vi "Find and assign COM Ports_1.vi"(8 "error in (no error)":errorcluster) -> (0 "error out":errorcluster, 2 "Available COM Ports":refnum<visa-resource-name>[](array[refnum]), 3 "Assigned VISA Ports":T1(array[cluster]))   [LabVIEW 2018]
uses:
  <vilib>/Instr/_visa.llb/VISA Find Search Mode.ctl
  <vilib>/Instr/_visa.llb/VISA Configure Serial Port (Instr).vi
panel:
  out "Available USB Ports":refnum<visa-resource-name>[](array[refnum])
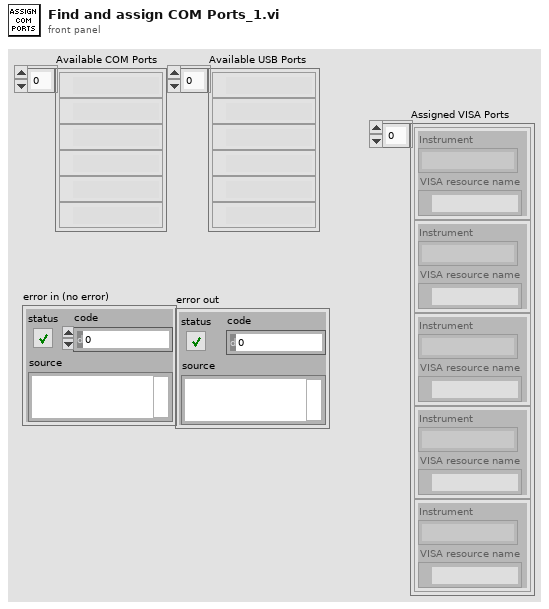
[diagram p1: front panel]
types:
  T1 = cluster{"Instrument":string, "VISA resource name":refnum<visa-resource-name>}[]
  T2 = enum16{"Switch", "SMU", "Vitrek", "Valhalla", "Stop"}
  T3 = typedef "VISA Find Search Mode.ctl" = u32
  T4 = cluster{"Instrument":string, "VISA resource name":refnum<visa-resource-name>}
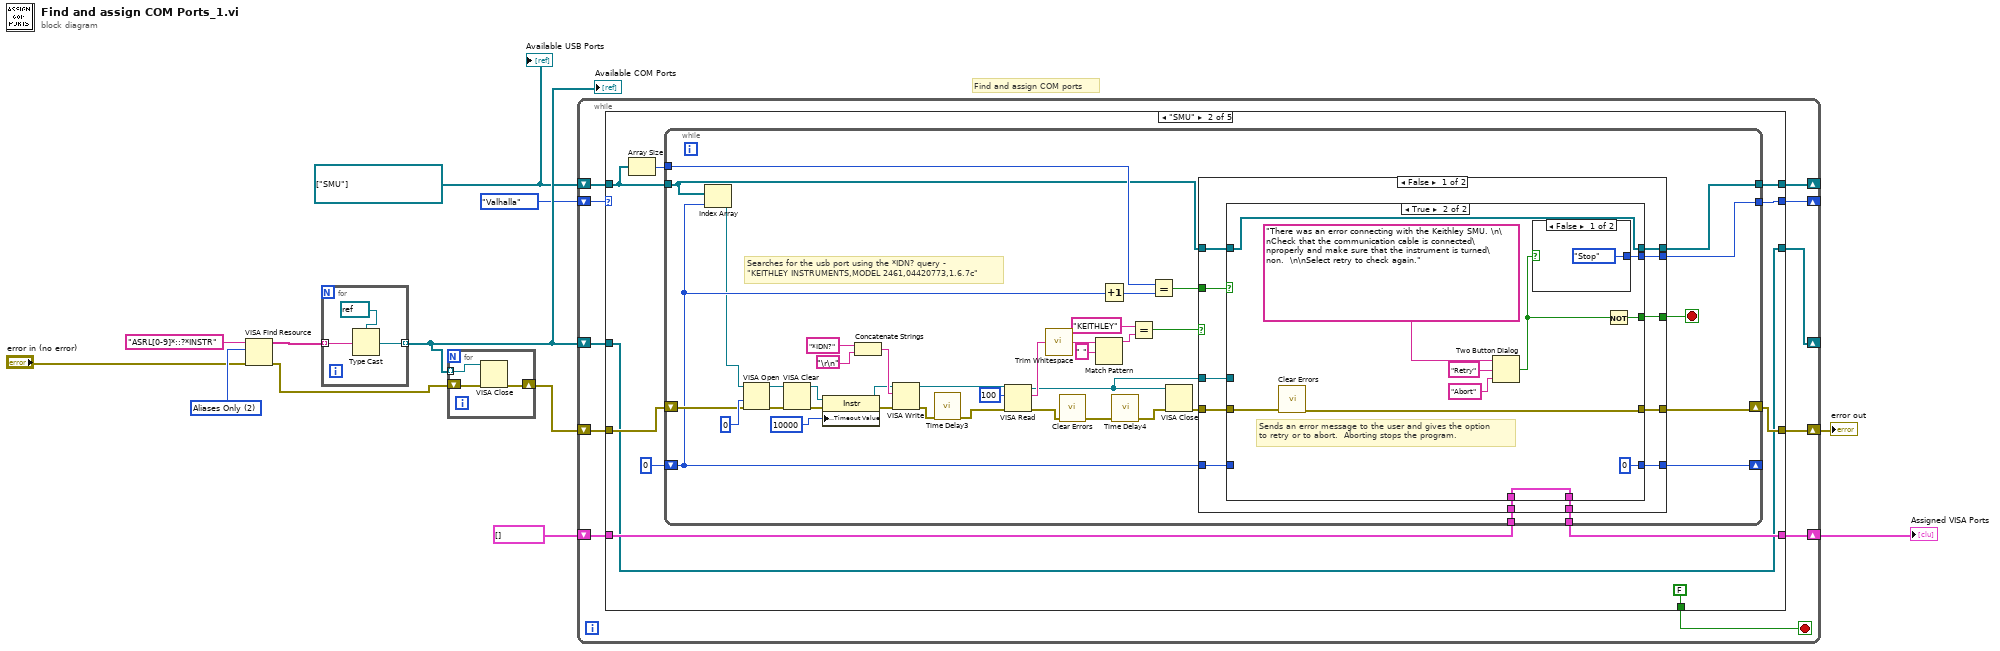
[diagram p0: block diagram]
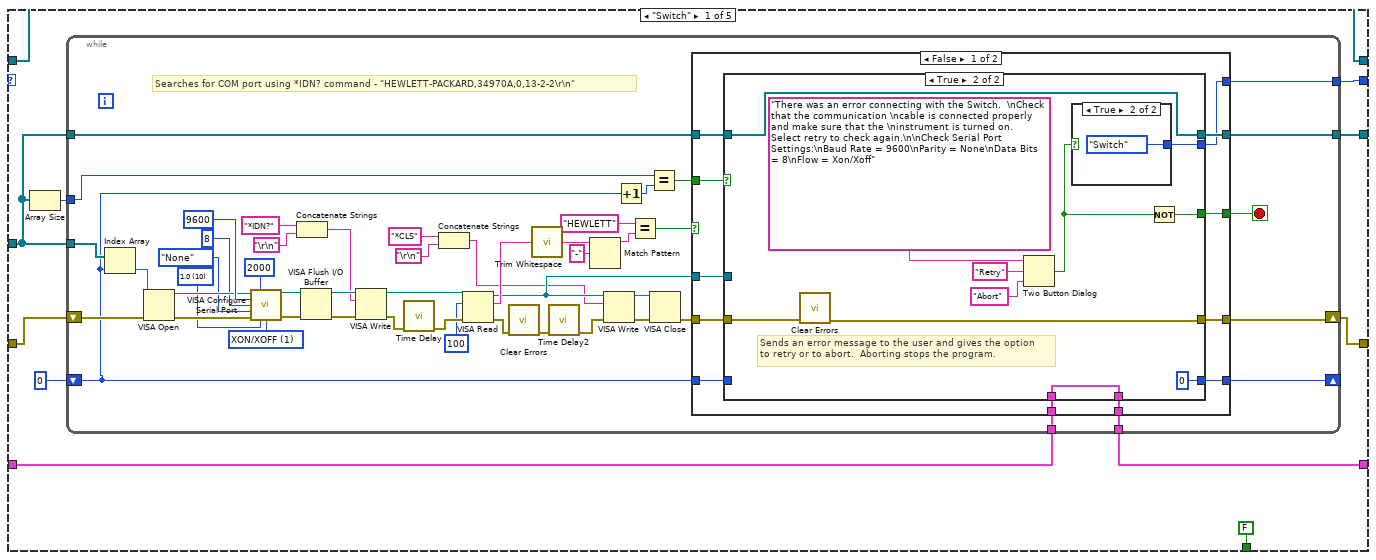
[diagram p2: hidden frame]
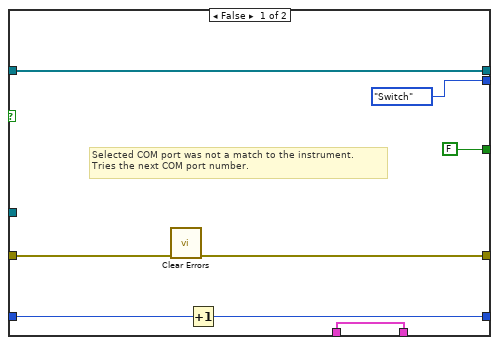
[diagram p3: hidden frame]
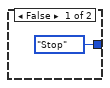
[diagram p4: hidden frame]
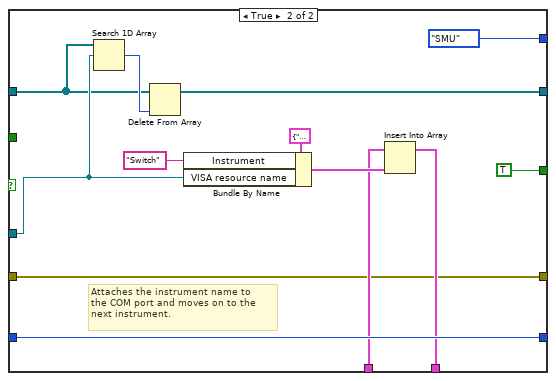
[diagram p5: hidden frame]
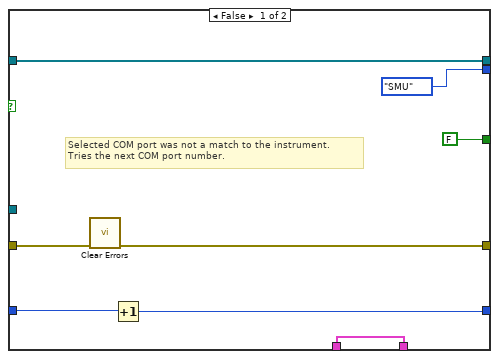
[diagram p6: hidden frame]
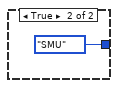
[diagram p7: hidden frame]
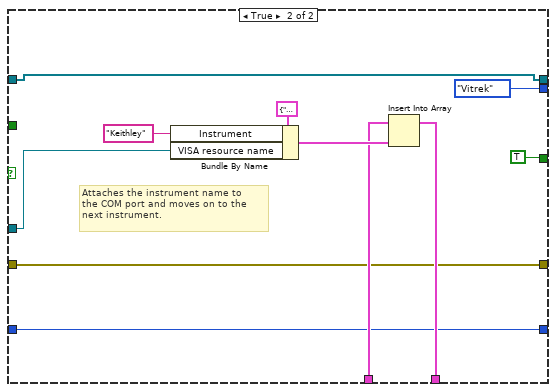
[diagram p8: hidden frame]
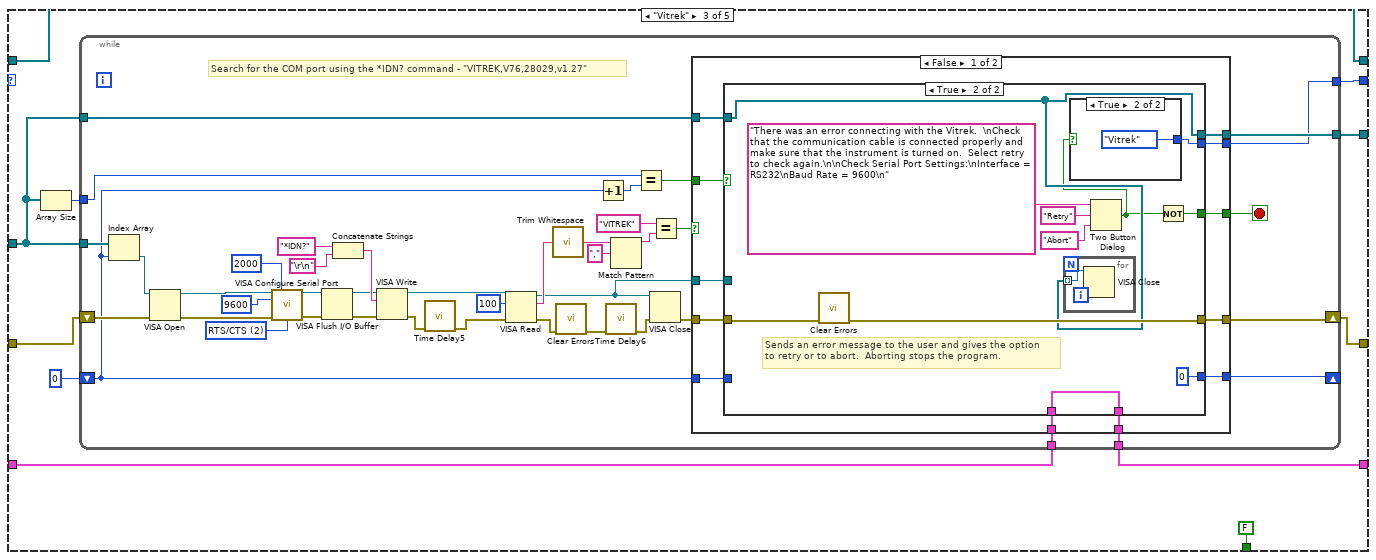
[diagram p9: hidden frame]
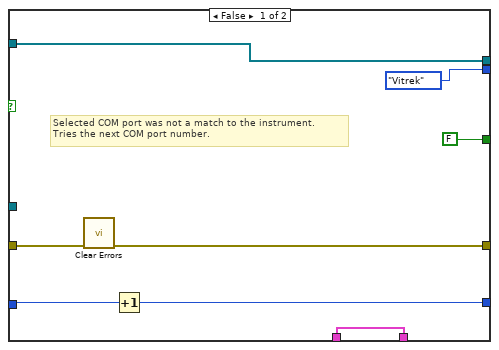
[diagram p10: hidden frame]
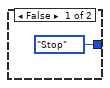
[diagram p11: hidden frame]
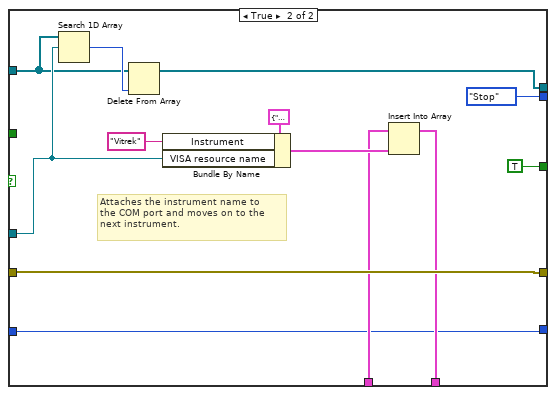
[diagram p12: hidden frame]
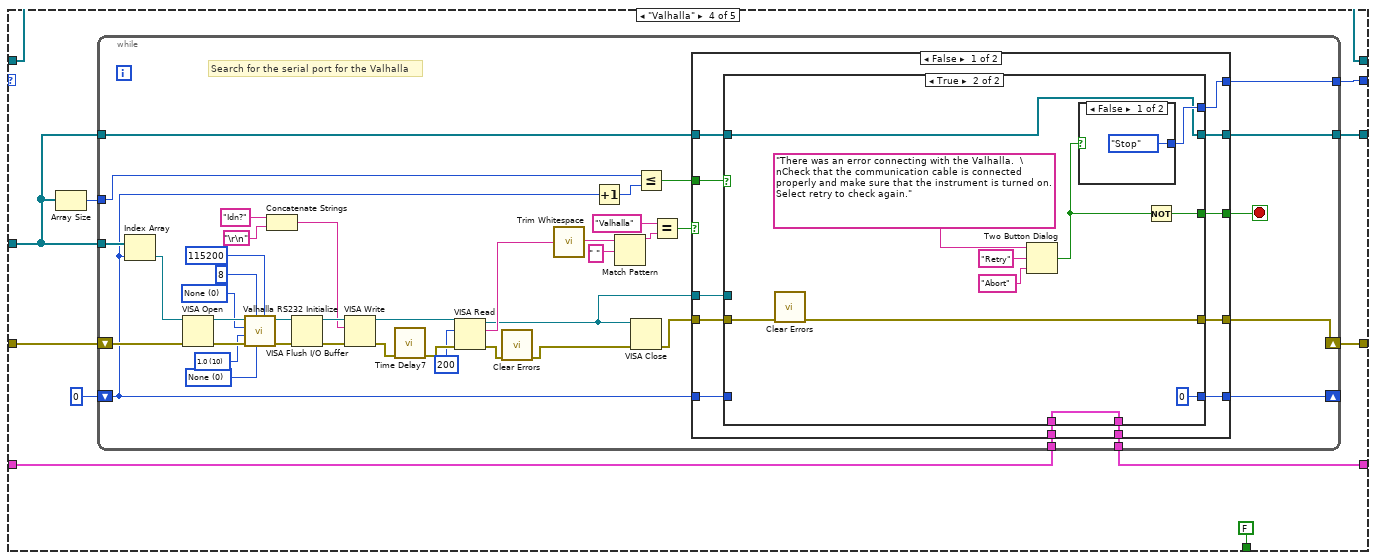
[diagram p13: hidden frame]
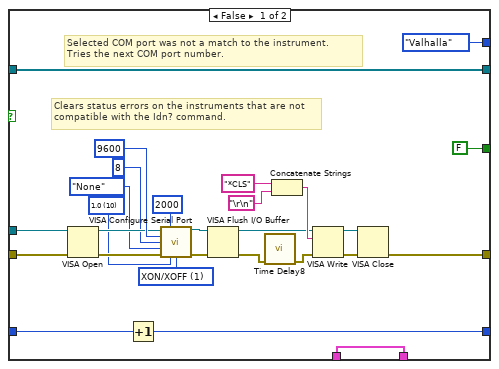
[diagram p14: hidden frame]
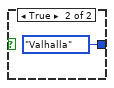
[diagram p15: hidden frame]
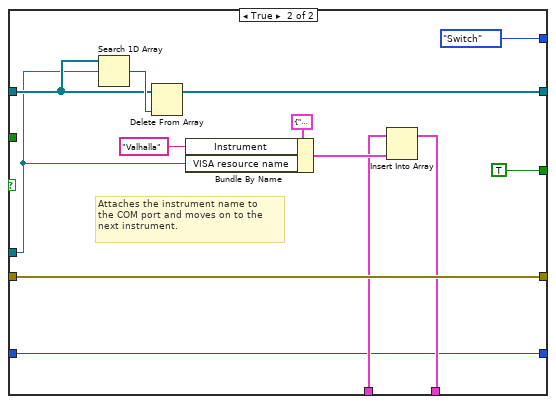
[diagram p16: hidden frame]
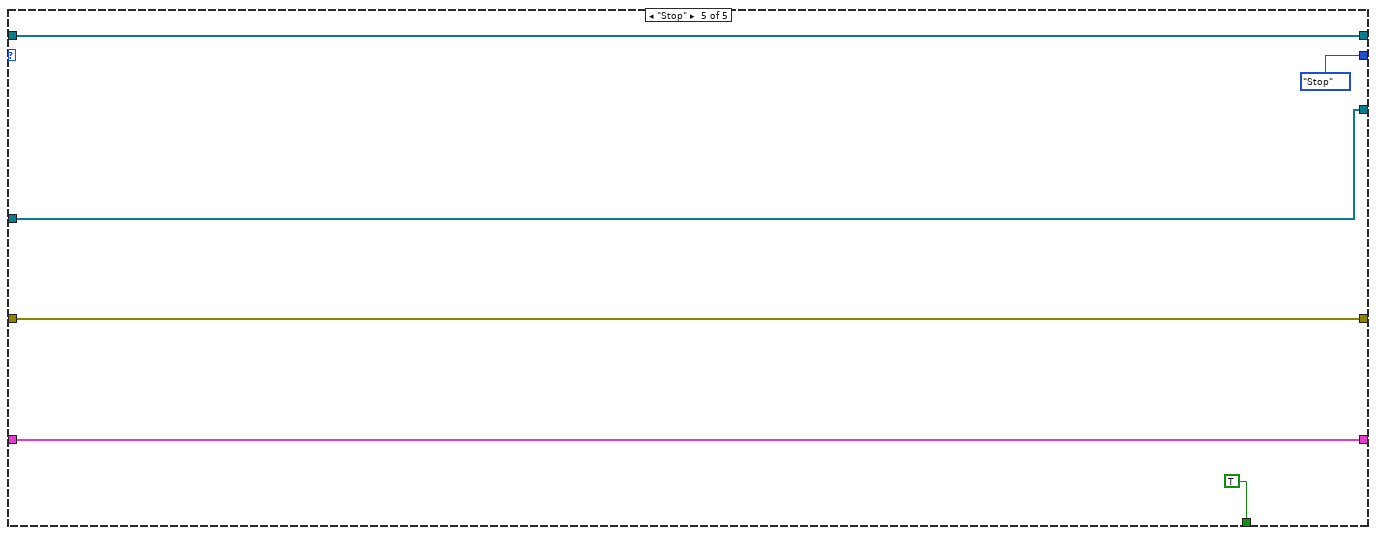
[diagram p17: hidden frame]
diagram:
  w1 = refnum<visa-resource-name>[] ["SMU"] ("Array")
  w7 = T3 2 items=["Canonical Names Only"=0, "Aliases Only"=2, "Include Matching Aliases"=3, "Include All Aliases"=4] ("Search Mode")
  # "Find and assign COM ports"
  n1 = VISA Find Resource(8:"error in (no error)", 10:w7, 11:"ASRL[0-9]*::?*INSTR" ("expression (\"?*\")")) -> (0:w3:errorcluster, 3:w8:string[])  [unwired: 1 out]
  n2 = for {
    tunnel: w8 -> [w14] mode=indexing
    tunnel: [w13] -> w12 mode=indexing
    n3 = Type Cast(type=refnum<visa-resource-name> refnum ("VISA resource name"), x=w14) -> (*(type *) &x=w13:refnum<visa-resource-name>)
  }
  "Available COM Ports" <- w12
  n4 = for {
    tunnel: w12 -> [w18] mode=indexing
    shift-right: [w16] -> w2
    shift-left: w3 -> [w17]
    n5 = VISA Close(VISA resource name=w18, error in (no error)=w17) -> (error out=w16:errorcluster)
  }
  n6 = while {
    shift-right: [w26] -> _
    shift-left: T2."Valhalla" ("Enum") -> [w28]
    shift-right: [w27] -> w11
    shift-left: T1 [] -> [w25]
    shift-right: [w24] -> _
    shift-left: w12 -> [w29]
    shift-right: [w22] -> w4
    shift-left: w2 -> [w23]
    shift-right: [w19] -> _
    shift-left: w1 -> [w20]
    stop <- w21 stop-if-true
    n7 = case shown="\"SMU\"" w28 {
      tunnel: [w33 w143 w235 w335 w456] -> w22
      tunnel: w29 -> [w37 w137 w239 w339 w454]
      tunnel: [w38 w146 w240 w340 w455] -> w27
      tunnel: [w35 w145 w237 w337 T2."Stop" ("Enum")] -> w26
      tunnel: w25 -> [w39 w147 w241 w341 w455]
      tunnel: [w36 w137 w238 w338 w454] -> w24
      tunnel: w23 -> [w34 w144 w236 w336 w456]
      tunnel: [FALSE FALSE FALSE FALSE TRUE] -> w21
      tunnel: w20 -> [w30 w140 w232 w332 w451]
      tunnel: [w30 w138 w232 w332 w451] -> w19
      frame "Switch" {
        n8 = Array Size(array=w37) -> (size(s)=w40:i32)
        n9 = while {
          tunnel: w37 -> [w46]
          tunnel: w40 -> [w81]
          tunnel: w39 -> [w72]
          tunnel: [w71] -> w38
          tunnel: w37 -> [w70]
          tunnel: [w69] -> w36
          tunnel: [w67] -> w35
          shift-right: [w66] -> w33
          shift-left: w34 -> [w65]
          shift-right: [w44] -> _
          shift-left: 0 -> [w41]
          stop <- w73 stop-if-true
          w60 = u16 10 items=["1.0"=10, "1.5"=15, "2.0"=20] ("stop bits (10: 1 bit)")
          w90 = u16 1 items=["None", "XON/XOFF", "RTS/CTS", "XON/XOFF & RTS/CTS", "DTR/DSR", "XON/XOFF & DTR/DSR"] ("flow control (0:none)")
          # "Searches for COM port using *IDN? command - \"HEWLETT-PACKARD,34970A,0,13-2-2\\r\\n\""
          n10 = Index Array(array=w46, index=w41) -> (element=w45:refnum<visa-resource-name>)
          n11 = VISA Open(error in (no error)=w65, VISA resource name=w45) -> (VISA resource name=w63:refnum<visa-resource-name>, error out=w64:errorcluster)  [unwired: 3 in]
          n12 = call-poly "VISA Configure Serial Port"("VISA resource name"=w63, "timeout (10sec)"=u32 2000, "baud rate (9600)"=u32 9600, "data bits (8)"=u16 8, "parity (0:none)"=enum16{"None", "Odd", "Even", "Mark", "Space"}."None", "error in (no error)"=w64, "stop bits (10: 1 bit)"=w60, "flow control (0:none)"=w90) -> ("VISA resource name out"=w77:refnum<visa-resource-name>, "error out"=w75:errorcluster)  [unwired: 6 in]
          n13 = Concatenate Strings("*IDN?" ("write buffer"), "\r\n") -> (w56:string)
          n14 = VISA Flush I/O Buffer(VISA resource name=w77, error in (no error)=w75) -> (VISA resource name out=w76:refnum<visa-resource-name>, error out=w74:errorcluster)  [unwired: 1 in]
          n15 = VISA Write(VISA resource name=w76, write buffer=w56, error in (no error)=w74) -> (VISA resource name out=w87:refnum<visa-resource-name>, error out=w88:errorcluster)  [unwired: 1 out]
          n16 = call "Time Delay"("error in (no error)"=w88) -> ("error out"=w86:errorcluster)  [unwired: 10 in]
          n17 = Concatenate Strings("*CLS" ("write buffer"), "\r\n") -> (w48:string)
          n18 = VISA Read(VISA resource name=w87, byte count=u32 100, error in (no error)=w86) -> (VISA resource name out=w50:refnum<visa-resource-name>, read buffer=w78:string, error out=w59:errorcluster)  [unwired: 1 out]
          n19 = call <vilib>:"Clear Errors.vi"("error in (no error)"=w59) -> ("error out"=w58:errorcluster)  [unwired: 5 in, 1 out]
          n20 = call <vilib>:"Trim Whitespace.vi"("string"=w78) -> ("trimmed string"=w80:string)  [unwired: 1 in]
          n21 = call "Time Delay2"("error in (no error)"=w58) -> ("error out"=w52:errorcluster)  [unwired: 10 in]
          n22 = Match Pattern(string=w80, regular expression="-") -> (before substring=w79:string)  [unwired: 1 in, 3 out]
          n23 = VISA Write(VISA resource name=w50, write buffer=w48, error in (no error)=w52) -> (VISA resource name out=w49:refnum<visa-resource-name>, error out=w51:errorcluster)  [unwired: 1 out]
          n24 = Increment(x=w41) -> (x+1=w47:i32)
          n25 = Equal?(x="HEWLETT", y=w79) -> (x = y?=w43:bool)
          n26 = Equal?(x=w81, y=w47) -> (x = y?=w42:bool)
          n27 = VISA Close(VISA resource name=w49, error in (no error)=w51) -> (error out=w68:errorcluster)
          n28 = case shown="False" w43 {
            tunnel: [w94 T2."SMU" ("Enum")] -> w67
            tunnel: [w95 TRUE] -> w73
            tunnel: w50 -> [w102 w128]
            tunnel: w72 -> [w101 w130]
            tunnel: [w100 w131] -> w71
            tunnel: w70 -> [w99 w127]
            tunnel: [w98 w125] -> w69
            tunnel: w68 -> [w97 w129]
            tunnel: [w96 w129] -> w66
            tunnel: w41 -> [w93 w132]
            tunnel: [w92 w132] -> w44
            tunnel: w42 -> [w91 _]
            frame False {
              n29 = case shown="True" w91 {
                tunnel: w102 -> [_ _]
                tunnel: w101 -> [w108 w111]
                tunnel: [w108 w111] -> w100
                tunnel: w99 -> [w110 w112]
                tunnel: [w110 w112] -> w98
                tunnel: w97 -> [w106 w116]
                tunnel: [w105 w115] -> w96
                tunnel: [FALSE w114] -> w95
                tunnel: [T2."Switch" ("Enum") w113] -> w94
                tunnel: w93 -> [w104 _]
                tunnel: [w103 0] -> w92
                frame False {
                  # "Selected COM port was not a match to the instrument.  \nTries the next COM port number."
                  n30 = call <vilib>:"Clear Errors.vi"("error in (no error)"=w106) -> ("error out"=w105:errorcluster)  [unwired: 5 in, 1 out]
                  n31 = Increment(x=w104) -> (x+1=w103:i32)
                }
                frame True {
                  # "Sends an error message to the user and gives the option\nto retry or to abort.  Aborting stops the program."
                  n32 = call <vilib>:"Clear Errors.vi"("error in (no error)"=w116) -> ("error out"=w115:errorcluster)  [unwired: 5 in, 1 out]
                  n33 = Two Button Dialog(message="There was an error connecting with the Switch.  \nCheck that the communication \ncable is connected properly and make sure that the \ninstrument is turned on.  Select retry to check again.\n\nCheck Serial Port Settings:\nBaud Rate = 9600\nParity = None\nData Bits = 8\nFlow = Xon/Xoff", 1:"Abort" ("F button name (\"Cancel\")"), 2:"Retry" ("T button name (\"OK\")")) -> (T button?=w117:bool)
                  n34 = case shown="True" w117 {
                    tunnel: [T2."Stop" ("Enum") T2."Switch" ("Enum")] -> w113
                    frame False {
                    }
                    frame True {
                    }
                  }
                  n35 = Not(x=w117) -> (.not. x?=w114:bool)
                }
              }
            }
            frame True {
              # "Attaches the instrument name to \nthe COM port and moves on to the\nnext instrument."
              n36 = Search 1D Array(1D array=w127, element=w128) -> (index of element=w136:i32)  [unwired: 1 in]
              n37 = Delete From Array(array=w127, index=w136) -> (array with subset deleted=w125:refnum<visa-resource-name>[])  [unwired: 1 in, 1 out]
              n38 = Bundle By Name(cluster=T4 {"Instrument"="", "VISA resource name"=""}, "Instrument"="Switch" ("x"), "VISA resource name"=w128) -> (w135:T4)
              n39 = Insert Into Array(array=w130, new element=w135) -> (w131:T1)  [unwired: 1 in]
            }
          }
        }
      }
      frame "SMU" {
        n40 = Array Size(array=w140) -> (size(s)=w139:i32)
        n41 = while {
          tunnel: w147 -> [w174]
          tunnel: [w173] -> w146
          tunnel: [w172] -> w145
          shift-right: [w171] -> w143
          shift-left: w144 -> [w165]
          shift-right: [w153] -> _
          shift-left: 0 -> [w152]
          tunnel: w140 -> [w149]
          tunnel: w139 -> [w150]
          tunnel: [w148] -> w138
          stop <- w175 stop-if-true
          # "Searches for the usb port using the *IDN? query - \n\"KEITHLEY INSTRUMENTS,MODEL 2461,04420773,1.6.7c\""
          n42 = Index Array(array=w149, index=w152) -> (element=w151:refnum<visa-resource-name>)
          n43 = VISA Open(access mode=u32 0, error in (no error)=w165, VISA resource name=w151) -> (VISA resource name=w164:refnum<visa-resource-name>, error out=w169:errorcluster)  [unwired: 2 out]
          n44 = VISA Clear(VISA resource name=w164, error in (no error)=w169) -> (VISA resource name out=w163:refnum<visa-resource-name>, error out=w170:errorcluster)
          n45 = property class="Instr"(reference=w163, error in=w170, "General Settings:Timeout Value"=u32 10000) -> (reference out=w162:refnum<visa-resource-name>, error out=w166:errorcluster)
          n46 = Concatenate Strings("*IDN?" ("write buffer"), "\r\n") -> (w186:string)
          n47 = VISA Write(VISA resource name=w162, write buffer=w186, error in (no error)=w166) -> (VISA resource name out=w183:refnum<visa-resource-name>, error out=w184:errorcluster)  [unwired: 1 out]
          n48 = call "Time Delay3"("error in (no error)"=w184) -> ("error out"=w182:errorcluster)  [unwired: 10 in]
          n49 = VISA Read(VISA resource name=w183, byte count=u32 100, error in (no error)=w182) -> (VISA resource name out=w160:refnum<visa-resource-name>, read buffer=w176:string, error out=w159:errorcluster)  [unwired: 1 out]
          n50 = call <vilib>:"Trim Whitespace.vi"("string"=w176) -> ("trimmed string"=w178:string)  [unwired: 1 in]
          n51 = call <vilib>:"Clear Errors.vi"("error in (no error)"=w159) -> ("error out"=w158:errorcluster)  [unwired: 5 in, 1 out]
          n52 = Match Pattern(string=w178, regular expression=" ") -> (before substring=w177:string)  [unwired: 1 in, 3 out]
          n53 = Increment(x=w152) -> (x+1=w154:i32)
          n54 = call "Time Delay4"("error in (no error)"=w158) -> ("error out"=w157:errorcluster)  [unwired: 10 in]
          n55 = Equal?(x="KEITHLEY", y=w177) -> (x = y?=w156:bool)
          n56 = Equal?(x=w150, y=w154) -> (x = y?=w155:bool)
          n57 = VISA Close(VISA resource name=w160, error in (no error)=w157) -> (error out=w161:errorcluster)
          n58 = case shown="False" w156 {
            tunnel: [w191 T2."Vitrek" ("Enum")] -> w172
            tunnel: [w192 TRUE] -> w175
            tunnel: w160 -> [w199 w223]
            tunnel: w174 -> [w198 w226]
            tunnel: [w197 w227] -> w173
            tunnel: w149 -> [w196 w224]
            tunnel: [w195 w224] -> w148
            tunnel: w161 -> [w194 w222]
            tunnel: [w193 w222] -> w171
            tunnel: w155 -> [w190 _]
            tunnel: w152 -> [w189 w221]
            tunnel: [w188 w221] -> w153
            frame False {
              n59 = case shown="True" w190 {
                tunnel: w199 -> [_ _]
                tunnel: w198 -> [w205 w209]
                tunnel: [w205 w209] -> w197
                tunnel: w196 -> [w207 w213]
                tunnel: [w207 w213] -> w195
                tunnel: w194 -> [w202 w214]
                tunnel: [w203 w210] -> w193
                tunnel: [FALSE w212] -> w192
                tunnel: [T2."SMU" ("Enum") w211] -> w191
                tunnel: w189 -> [w201 _]
                tunnel: [w200 0] -> w188
                frame False {
                  # "Selected COM port was not a match to the instrument.  \nTries the next COM port number."
                  n60 = call <vilib>:"Clear Errors.vi"("error in (no error)"=w202) -> ("error out"=w203:errorcluster)  [unwired: 5 in, 1 out]
                  n61 = Increment(x=w201) -> (x+1=w200:i32)
                }
                frame True {
                  # "Sends an error message to the user and gives the option\nto retry or to abort.  Aborting stops the program."
                  n62 = call <vilib>:"Clear Errors.vi"("error in (no error)"=w214) -> ("error out"=w210:errorcluster)  [unwired: 5 in, 1 out]
                  n63 = Two Button Dialog(message="There was an error connecting with the Keithley SMU. \n\nCheck that the communication cable is connected\nproperly and make sure that the instrument is turned\non.  \n\nSelect retry to check again.", 1:"Abort" ("F button name (\"Cancel\")"), 2:"Retry" ("T button name (\"OK\")")) -> (T button?=w215:bool)
                  n64 = case shown="False" w215 {
                    tunnel: [T2."Stop" ("Enum") T2."SMU" ("Enum")] -> w211
                    frame False {
                    }
                    frame True {
                    }
                  }
                  n65 = Not(x=w215) -> (.not. x?=w212:bool)
                }
              }
            }
            frame True {
              # "Attaches the instrument name to \nthe COM port and moves on to the\nnext instrument."
              n66 = Bundle By Name(cluster=T4 {"Instrument"="", "VISA resource name"=""}, "Instrument"="Keithley" ("x"), "VISA resource name"=w223) -> (w231:T4)
              n67 = Insert Into Array(array=w226, new element=w231) -> (w227:T1)  [unwired: 1 in]
            }
          }
        }
      }
      frame "Vitrek" {
        n68 = Array Size(array=w239) -> (size(s)=w242:i32)
        n69 = while {
          tunnel: w239 -> [w249]
          tunnel: w242 -> [w272]
          tunnel: w241 -> [w263]
          tunnel: [w262] -> w240
          tunnel: w239 -> [w261]
          tunnel: [w260] -> w238
          tunnel: [w258] -> w237
          shift-right: [w257] -> w235
          shift-left: w236 -> [w255]
          shift-right: [w246] -> _
          shift-left: 0 -> [w243]
          stop <- w264 stop-if-true
          w284 = u16 2 items=["None", "XON/XOFF", "RTS/CTS", "XON/XOFF & RTS/CTS", "DTR/DSR", "XON/XOFF & DTR/DSR"] ("flow control (0:none)")
          # "Search for the COM port using the *IDN? command - \"VITREK,V76,28029,v1.27\""
          n70 = Index Array(array=w249, index=w243) -> (element=w248:refnum<visa-resource-name>)
          n71 = VISA Open(error in (no error)=w255, VISA resource name=w248) -> (VISA resource name=w253:refnum<visa-resource-name>, error out=w254:errorcluster)  [unwired: 3 in]
          n72 = call-poly "VISA Configure Serial Port"("VISA resource name"=w253, "timeout (10sec)"=u32 2000, "baud rate (9600)"=u32 9600, "error in (no error)"=w254, "flow control (0:none)"=w284) -> ("VISA resource name out"=w268:refnum<visa-resource-name>, "error out"=w266:errorcluster)  [unwired: 9 in]
          n73 = VISA Flush I/O Buffer(VISA resource name=w268, error in (no error)=w266) -> (VISA resource name out=w267:refnum<visa-resource-name>, error out=w265:errorcluster)  [unwired: 1 in]
          n74 = Concatenate Strings("*IDN?" ("write buffer"), "\r\n") -> (w281:string)
          n75 = VISA Write(VISA resource name=w267, write buffer=w281, error in (no error)=w265) -> (VISA resource name out=w278:refnum<visa-resource-name>, error out=w279:errorcluster)  [unwired: 1 out]
          n76 = call "Time Delay5"("error in (no error)"=w279) -> ("error out"=w277:errorcluster)  [unwired: 10 in]
          n77 = VISA Read(VISA resource name=w278, byte count=u32 100, error in (no error)=w277) -> (VISA resource name out=w256:refnum<visa-resource-name>, read buffer=w269:string, error out=w252:errorcluster)  [unwired: 1 out]
          n78 = call <vilib>:"Trim Whitespace.vi"("string"=w269) -> ("trimmed string"=w271:string)  [unwired: 1 in]
          n79 = call <vilib>:"Clear Errors.vi"("error in (no error)"=w252) -> ("error out"=w251:errorcluster)  [unwired: 5 in, 1 out]
          n80 = Increment(x=w243) -> (x+1=w247:i32)
          n81 = call "Time Delay6"("error in (no error)"=w251) -> ("error out"=w250:errorcluster)  [unwired: 10 in]
          n82 = Match Pattern(string=w271, regular expression=",") -> (before substring=w270:string)  [unwired: 1 in, 3 out]
          n83 = Equal?(x=w272, y=w247) -> (x = y?=w244:bool)
          n84 = VISA Close(VISA resource name=w256, error in (no error)=w250) -> (error out=w259:errorcluster)
          n85 = Equal?(x="VITREK", y=w270) -> (x = y?=w245:bool)
          n86 = case shown="False" w245 {
            tunnel: [w288 T2."Stop" ("Enum")] -> w258
            tunnel: [w289 TRUE] -> w264
            tunnel: w256 -> [w296 w327]
            tunnel: w263 -> [w295 w323]
            tunnel: [w294 w322] -> w262
            tunnel: w261 -> [w293 w320]
            tunnel: [w292 w321] -> w260
            tunnel: w259 -> [w291 w324]
            tunnel: [w290 w324] -> w257
            tunnel: w243 -> [w287 w319]
            tunnel: [w286 w319] -> w246
            tunnel: w244 -> [w285 _]
            frame False {
              n87 = case shown="True" w285 {
                tunnel: w296 -> [_ _]
                tunnel: w295 -> [w302 w308]
                tunnel: [w302 w308] -> w294
                tunnel: w293 -> [w304 w309]
                tunnel: [w304 w309] -> w292
                tunnel: w291 -> [w299 w312]
                tunnel: [w300 w311] -> w290
                tunnel: [FALSE w307] -> w289
                tunnel: [T2."Vitrek" ("Enum") w310] -> w288
                tunnel: w287 -> [w298 _]
                tunnel: [w297 0] -> w286
                frame False {
                  # "Selected COM port was not a match to the instrument.  \nTries the next COM port number."
                  n88 = call <vilib>:"Clear Errors.vi"("error in (no error)"=w299) -> ("error out"=w300:errorcluster)  [unwired: 5 in, 1 out]
                  n89 = Increment(x=w298) -> (x+1=w297:i32)
                }
                frame True {
                  # "Sends an error message to the user and gives the option\nto retry or to abort.  Aborting stops the program."
                  n90 = call <vilib>:"Clear Errors.vi"("error in (no error)"=w312) -> ("error out"=w311:errorcluster)  [unwired: 5 in, 1 out]
                  n91 = for {
                    tunnel: w309 -> [w318] mode=indexing
                    n92 = VISA Close(VISA resource name=w318) -> ()  [unwired: 1 in, 1 out]
                  }
                  n93 = Two Button Dialog(message="There was an error connecting with the Vitrek.  \nCheck that the communication cable is connected properly and make sure that the instrument is turned on.  Select retry to check again.\n\nCheck Serial Port Settings:\nInterface = RS232\nBaud Rate = 9600\n", 1:"Abort" ("F button name (\"Cancel\")"), 2:"Retry" ("T button name (\"OK\")")) -> (T button?=w306:bool)
                  n94 = case shown="True" w306 {
                    tunnel: [T2."Stop" ("Enum") T2."Vitrek" ("Enum")] -> w310
                    frame False {
                    }
                    frame True {
                    }
                  }
                  n95 = Not(x=w306) -> (.not. x?=w307:bool)
                }
              }
            }
            frame True {
              # "Attaches the instrument name to \nthe COM port and moves on to the\nnext instrument."
              n96 = Search 1D Array(1D array=w320, element=w327) -> (index of element=w331:i32)  [unwired: 1 in]
              n97 = Delete From Array(array=w320, index=w331) -> (array with subset deleted=w321:refnum<visa-resource-name>[])  [unwired: 1 in, 1 out]
              n98 = Bundle By Name(cluster=T4 {"Instrument"="", "VISA resource name"=""}, "Instrument"="Vitrek" ("x"), "VISA resource name"=w327) -> (w330:T4)
              n99 = Insert Into Array(array=w323, new element=w330) -> (w322:T1)  [unwired: 1 in]
            }
          }
        }
      }
      frame "Valhalla" {
        n100 = Array Size(array=w339) -> (size(s)=w342:i32)
        n101 = while {
          tunnel: w339 -> [w346]
          tunnel: w342 -> [w385]
          tunnel: w341 -> [w383]
          tunnel: [w382] -> w340
          tunnel: w339 -> [w381]
          tunnel: [w380] -> w338
          tunnel: [w379] -> w337
          shift-right: [w378] -> w335
          shift-left: w336 -> [w355]
          shift-right: [w347] -> _
          shift-left: 0 -> [w343]
          stop <- w384 stop-if-true
          w357 = u16 10 items=["1.0"=10, "1.5"=15, "2.0"=20] ("Stop Bits")
          w356 = u16 0 items=["None", "Odd", "Even", "Mark", "Space"] ("Parity")
          w359 = u16 0 items=["None", "XON/XOFF", "RTS/CTS", "XON/XOFF & RTS/CTS", "DTR/DSR", "XON/XOFF & DTR/DSR"] ("Flow Control")
          # "Search for the serial port for the Valhalla"
          n102 = Index Array(array=w346, index=w343) -> (element=w345:refnum<visa-resource-name>)
          n103 = VISA Open(error in (no error)=w355, VISA resource name=w345) -> (VISA resource name=w370:refnum<visa-resource-name>, error out=w371:errorcluster)  [unwired: 3 in]
          n104 = call "Valhalla RS232 Initialize.vi"("Baud Rate"=u32 115200, "Flow Control"=w359, "Data Bits"=u16 8, "error in (no error)"=w371, "Stop Bits"=w357, "Parity"=w356, "VISA Refnum in"=w370) -> ("error out"=w373:errorcluster, "VISA Refnum out"=w372:refnum<visa-resource-name>)  [unwired: 3 in]
          n105 = Concatenate Strings("Idn?" ("write buffer"), "\r\n") -> (w364:string)
          n106 = VISA Flush I/O Buffer(VISA resource name=w372, error in (no error)=w373) -> (VISA resource name out=w369:refnum<visa-resource-name>, error out=w368:errorcluster)  [unwired: 1 in]
          n107 = VISA Write(VISA resource name=w369, write buffer=w364, error in (no error)=w368) -> (VISA resource name out=w366:refnum<visa-resource-name>, error out=w365:errorcluster)  [unwired: 1 out]
          n108 = call "Time Delay7"("error in (no error)"=w365) -> ("error out"=w367:errorcluster)  [unwired: 10 in]
          n109 = VISA Read(VISA resource name=w366, byte count=u32 200, error in (no error)=w367) -> (VISA resource name out=w351:refnum<visa-resource-name>, read buffer=w354:string, error out=w352:errorcluster)  [unwired: 1 out]
          n110 = call <vilib>:"Clear Errors.vi"("error in (no error)"=w352) -> ("error out"=w350:errorcluster)  [unwired: 5 in, 1 out]
          n111 = call <vilib>:"Trim Whitespace.vi"("string"=w354) -> ("trimmed string"=w375:string)  [unwired: 1 in]
          n112 = Increment(x=w343) -> (x+1=w344:i32)
          n113 = Match Pattern(string=w375, regular expression=" ") -> (before substring=w374:string)  [unwired: 1 in, 3 out]
          n114 = VISA Close(VISA resource name=w351, error in (no error)=w350) -> (error out=w353:errorcluster)
          n115 = Less Or Equal?(x=w385, y=w344) -> (x <= y?=w349:bool)
          n116 = Equal?(x="Valhalla", y=w374) -> (x = y?=w348:bool)
          n117 = case shown="False" w348 {
            tunnel: [w389 T2."Switch" ("Enum")] -> w379
            tunnel: [w390 TRUE] -> w384
            tunnel: w351 -> [w397 w445]
            tunnel: w383 -> [w396 w443]
            tunnel: [w395 w439] -> w382
            tunnel: w381 -> [w394 w446]
            tunnel: [w393 w442] -> w380
            tunnel: w353 -> [w392 w444]
            tunnel: [w391 w444] -> w378
            tunnel: w349 -> [w388 _]
            tunnel: w343 -> [w387 w438]
            tunnel: [w386 w438] -> w347
            frame False {
              n118 = case shown="True" w388 {
                tunnel: w397 -> [w419 _]
                tunnel: w396 -> [w422 w426]
                tunnel: [w422 w426] -> w395
                tunnel: w394 -> [w424 w427]
                tunnel: [w424 w427] -> w393
                tunnel: w392 -> [w420 w431]
                tunnel: [w418 w429] -> w391
                tunnel: [FALSE w430] -> w390
                tunnel: [T2."Valhalla" ("Enum") w428] -> w389
                tunnel: w387 -> [w399 _]
                tunnel: [w398 0] -> w386
                frame False {
                  w407 = u16 10 items=["1.0"=10, "1.5"=15, "2.0"=20] ("stop bits (10: 1 bit)")
                  w414 = u16 1 items=["None", "XON/XOFF", "RTS/CTS", "XON/XOFF & RTS/CTS", "DTR/DSR", "XON/XOFF & DTR/DSR"] ("flow control (0:none)")
                  # "Clears status errors on the instruments that are not\ncompatible with the Idn? command."
                  # "Selected COM port was not a match to the instrument.  \nTries the next COM port number."
                  n119 = VISA Open(error in (no error)=w420, VISA resource name=w419) -> (VISA resource name=w410:refnum<visa-resource-name>, error out=w411:errorcluster)  [unwired: 3 in]
                  n120 = Increment(x=w399) -> (x+1=w398:i32)
                  n121 = call-poly "VISA Configure Serial Port"("VISA resource name"=w410, "timeout (10sec)"=u32 2000, "baud rate (9600)"=u32 9600, "data bits (8)"=u16 8, "parity (0:none)"=enum16{"None", "Odd", "Even", "Mark", "Space"}."None", "error in (no error)"=w411, "stop bits (10: 1 bit)"=w407, "flow control (0:none)"=w414) -> ("VISA resource name out"=w404:refnum<visa-resource-name>, "error out"=w402:errorcluster)  [unwired: 6 in]
                  n122 = VISA Flush I/O Buffer(VISA resource name=w404, error in (no error)=w402) -> (VISA resource name out=w403:refnum<visa-resource-name>, error out=w401:errorcluster)  [unwired: 1 in]
                  n123 = call "Time Delay8"("error in (no error)"=w401) -> ("error out"=w400:errorcluster)  [unwired: 10 in]
                  n124 = Concatenate Strings("*CLS" ("write buffer"), "\r\n") -> (w415:string)
                  n125 = VISA Write(VISA resource name=w403, write buffer=w415, error in (no error)=w400) -> (VISA resource name out=w405:refnum<visa-resource-name>, error out=w406:errorcluster)  [unwired: 1 out]
                  n126 = VISA Close(VISA resource name=w405, error in (no error)=w406) -> (error out=w418:errorcluster)
                }
                frame True {
                  n127 = call <vilib>:"Clear Errors.vi"("error in (no error)"=w431) -> ("error out"=w429:errorcluster)  [unwired: 5 in, 1 out]
                  n128 = Two Button Dialog(message="There was an error connecting with the Valhalla.  \nCheck that the communication cable is connected properly and make sure that the instrument is turned on.  Select retry to check again.", 1:"Abort" ("F button name (\"Cancel\")"), 2:"Retry" ("T button name (\"OK\")")) -> (T button?=w432:bool)
                  n129 = case shown="False" w432 {
                    tunnel: [T2."Stop" ("Enum") T2."Valhalla" ("Enum")] -> w428
                    frame False {
                    }
                    frame True {
                    }
                  }
                  n130 = Not(x=w432) -> (.not. x?=w430:bool)
                }
              }
            }
            frame True {
              # "Attaches the instrument name to \nthe COM port and moves on to the\nnext instrument."
              n131 = Search 1D Array(1D array=w446, element=w445) -> (index of element=w450:i32)  [unwired: 1 in]
              n132 = Delete From Array(array=w446, index=w450) -> (array with subset deleted=w442:refnum<visa-resource-name>[])  [unwired: 1 in, 1 out]
              n133 = Bundle By Name(cluster=T4 {"Instrument"="", "VISA resource name"=""}, "Instrument"="Valhalla" ("x"), "VISA resource name"=w445) -> (w449:T4)
              n134 = Insert Into Array(array=w443, new element=w449) -> (w439:T1)  [unwired: 1 in]
            }
          }
        }
      }
      frame "Stop" {
      }
    }
  }
  "Assigned VISA Ports" <- w11
  "error out" <- w4
  "Available USB Ports" <- w1
